vi "Example_Demo.vi"() -> ()   [LabVIEW 2017, in "maxonEPOS.lvlib"]
doc: "Example how to work with some maxon EPOS VIs. Before starts this example the device must be tuned and the parameter settings must be correct.\nThe example shows:\n - how to initialise and close an interface (with a dialog)\n - dialog shows configured parameters and data\n - enable/disable a device\n - start/stop a relative movement\n - profile and node settings\n - use of the data recorder\n - update of actual values\n\nThe example must be terminated with the button \"Exit\"!"
uses:
  maxonEPOS.lvlib
panel:
  in  "data recorder":T1={"samplingPeriod"=12, "nbOfPrecedingSamples"=0}
  out "Position Graph":i32[](graph)=[374267, 374268, 374268, 374269, 374271, 374273, 374275, 374279, 374282, 374287, 374291, 374296, 374301, 374306, 374311, 374317, 374322, 374327, 374333, 374340, 374347, 374354, 374362, 374371, 374380, 374390, 374399, 374408, 374417, 374428, 374438, 374450, 374461, 374471, 374482, 374492, 374504, 374517, 374531, 374545, 374560, 374574, 374589, 374604, 374620, 374635, 374649, 374665, 374682, 374699, 374716, 374732, 374751, 374769, 374787, 374806, 374825, 374843, 374860, 374874, 374886, 374898, 374910, 374922, 374934, 374946, 374958, 374969, 374982, 374996, 375011, 375023, 375035, 375046, 375056, 375066, 375076, 375085, 375093, 375102, 375110, 375119, 375128, 375137, 375146, 375154, 375162, 375169, 375175, 375181, 375187, 375191, 375197, 375201, 375206, 375211, 375215, 375219, 375224, 375227, 375231, 375233, 375236, 375237, 375239, 375240, 375240, 375241, 375241, 375241, 375241, 375241, 375241, 375242, 375243, 375244, 375245, 375247, 375248, 375250, 375251, 375252, 375253, 375254, 375255, 375256, 375256, 375257, 375257, 375257, 375257, 375258, 375258, 375259, 375259, 375260, 375261, 375261, 375262, 375262, 375263, 375263, 375263, 375263, 375264, 375264, 375264, 375265, 375265, 375265, 375266, 375266, 375266, 375266, 375266, 375267, 375267, 375267, 375267, 375267, 375267, 375267, 375267, 375267, 375268, 375268, 375268, 375268, 375268, 375268, 375268, 375268, 375268, 375268, 375268, 375268, 375268, 375268, 375268, 375268, 375268, 375268, 375268, 375268, 375268, 375268, 375268, 375268, 375268, 375268, 375268, 375268, 375268, 375268, 375268, 375268, 375268, 375268, 375268, 375268, 375268, 375268, 375268, 375268, 375268, 375268, 375268, 375268, 375268, 375268, 375268, 375268, 375268, 375268, 375268, 375268, 375268, 375268, 375268, 375268, 375268, 375268, 375268, 375268, 375268, 375268, 375268, 375268, 375268, 375268, 375268, 375268, 375268, 375268, 375268, 375268, 375268, 375268, 375268, 375268, 375268, 375268, 375268, 375268, 375268, 375268, 375268, 375268, 375268, 375268, 375268, 375268, 375268, 375268, 375268, 375268]
  in  "flags":cluster{"Absolute":i32, "Immediately":i32}={"Absolute"=0, "Immediately"=1} {"Immediately" items=["false", "true"]; "Absolute" items=["false", "true"]}
  out "axis data ex":T2
  out "enabled":bool=TRUE
  in  "Exit":bool
  in  "relative position":i32=1000
  in  "position profile":T3={"profileVelocity"=1000, "profileAcceleration"=10000, "profileDeceleration"=10000}
  in  "nodeId":u16=1
  in  "ShowParameters":bool
  in  "DeviceSettings":bool
  in  "MoveToPosition":bool
  in  "Halt":bool
  in  "Enable / Disable":bool
  in  "Axis":cluster{"keyHandle":u32, "nodeId":u16}
  # "EPOS2/4 Positioning Demo"
  # "Position Profile"
  # "Actual Values"
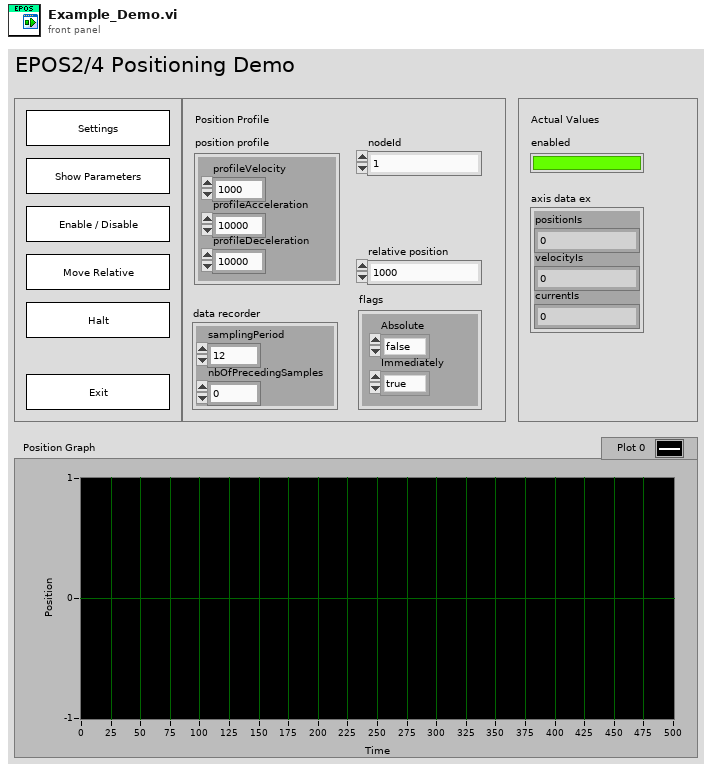
[diagram p1: front panel]
types:
  T1 = cluster{"samplingPeriod":u16, "nbOfPrecedingSamples":u16}
  T2 = cluster{"positionIs":i32, "velocityIs":i32, "currentIs":i32}
  T3 = cluster{"profileVelocity":u32, "profileAcceleration":u32, "profileDeceleration":u32}
  T4 = cluster{"Enum":enum16{"Device Settings", "Halt", "Move Position", "ShowParameters", "Enable-Disable", "Exit", "Update"}, bool}
  T5 = cluster{"recorded object 1":cluster{"objectIndex":u16, "objectSubIndex":u8, "objectSize":u8}, "recorded object 2":cluster{"objectIndex":u16, "objectSubIndex":u8, "objectSize":u8}, "recorded object 3":cluster{"objectIndex":u16, "objectSubIndex":u8, "objectSize":u8}, "recorded object 4":cluster{"objectIndex":u16, "objectSubIndex":u8, "objectSize":u8}}
  T6 = enum16{"Disabled", "Enabled", "Quickstop", "Fault"}
  T7 = enum16{"Device Settings", "Halt", "Move Position", "ShowParameters", "Enable-Disable", "Exit", "Update"}
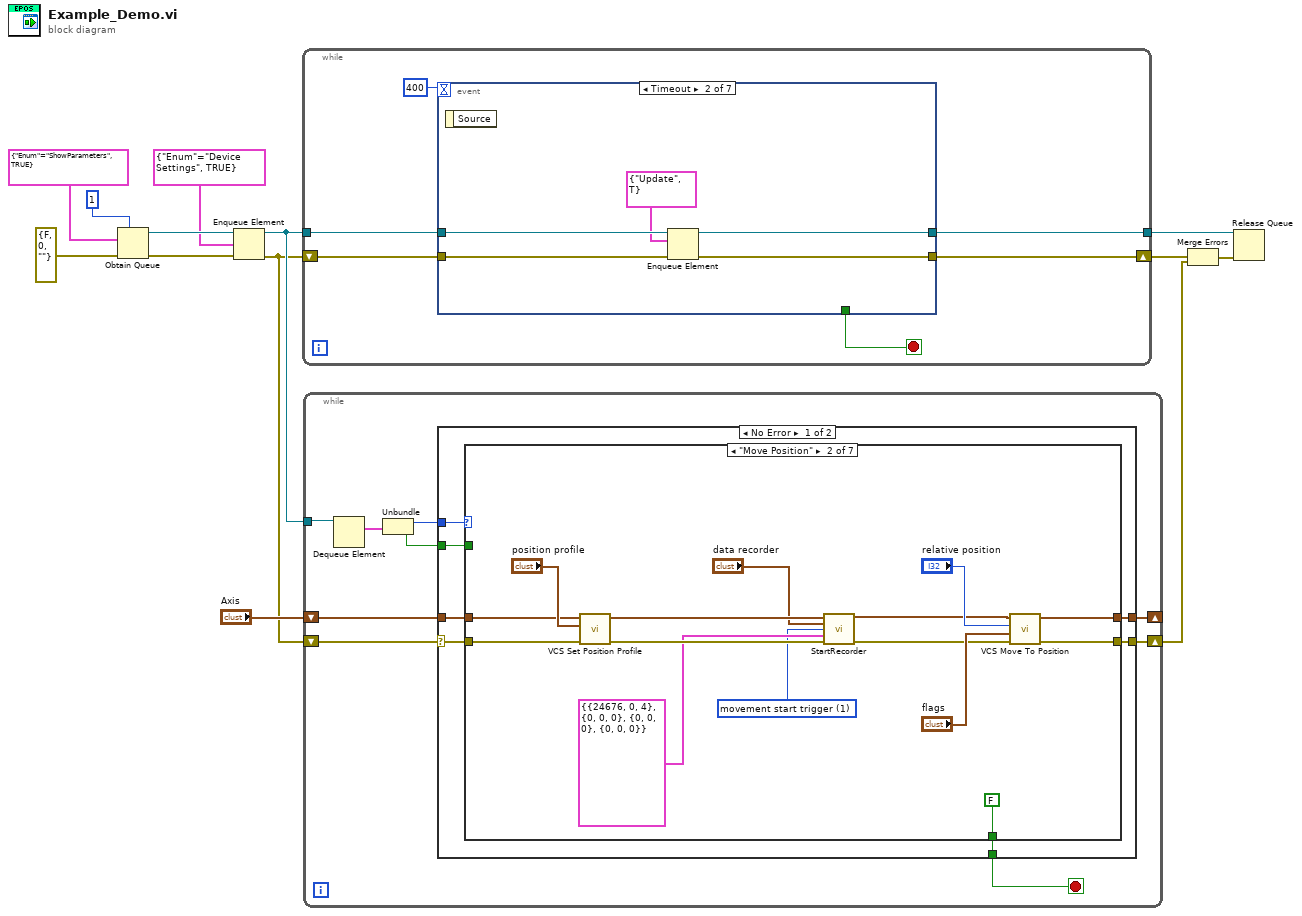
[diagram p0: block diagram]
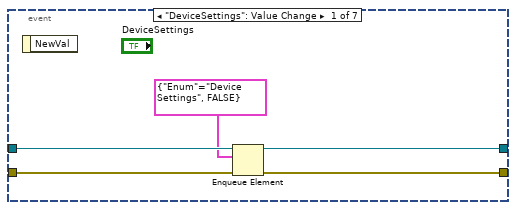
[diagram p2: hidden frame]
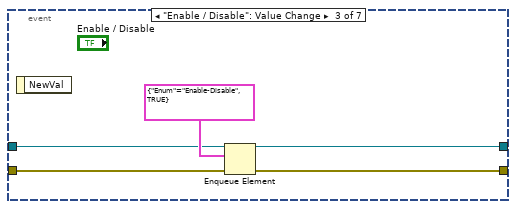
[diagram p3: hidden frame]
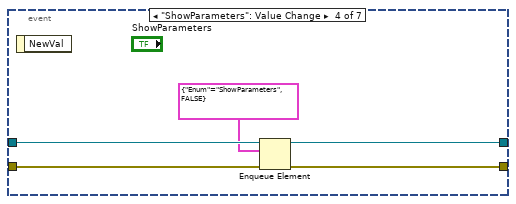
[diagram p4: hidden frame]
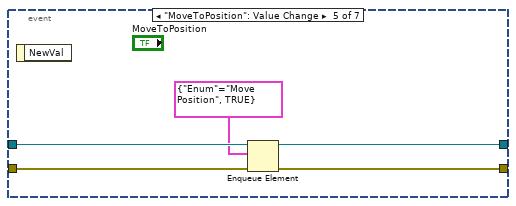
[diagram p5: hidden frame]
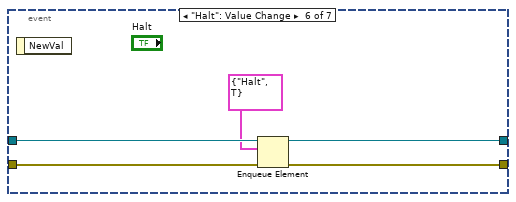
[diagram p6: hidden frame]
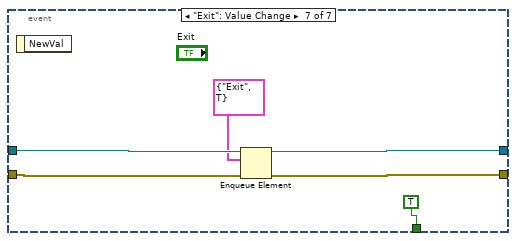
[diagram p7: hidden frame]
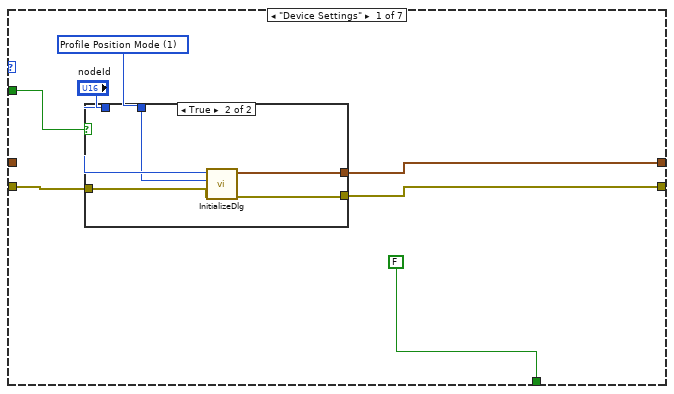
[diagram p8: hidden frame]
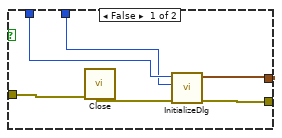
[diagram p9: hidden frame]
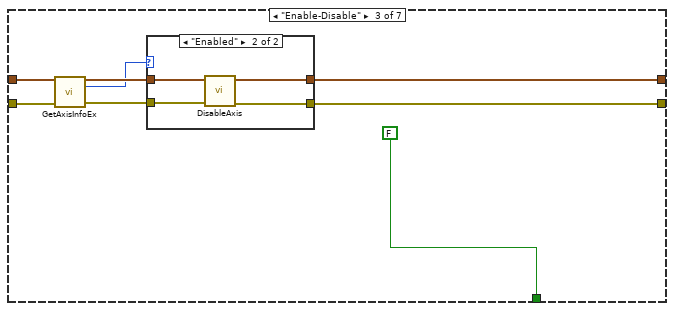
[diagram p10: hidden frame]
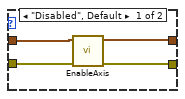
[diagram p11: hidden frame]
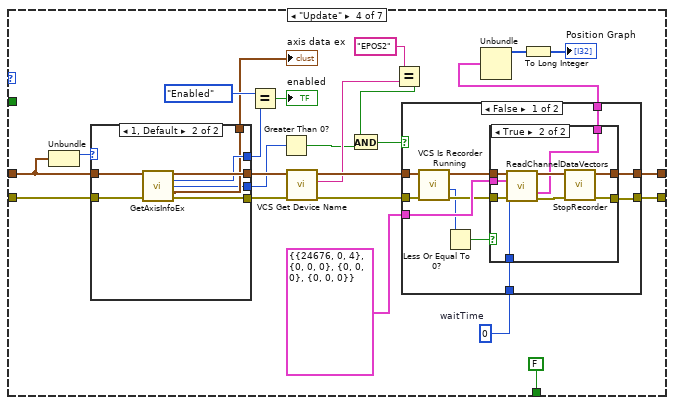
[diagram p12: hidden frame]
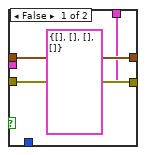
[diagram p13: hidden frame]
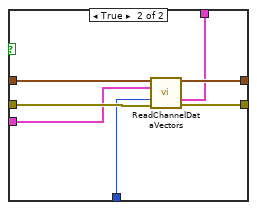
[diagram p14: hidden frame]
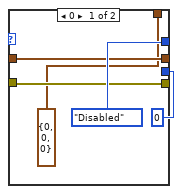
[diagram p15: hidden frame]
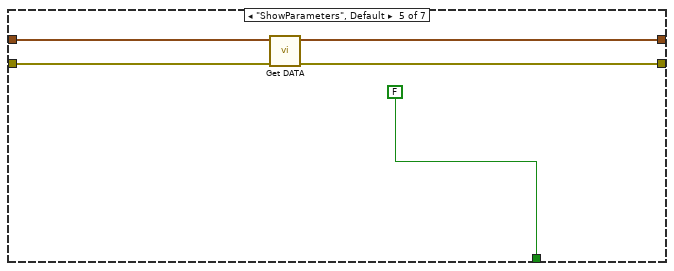
[diagram p16: hidden frame]
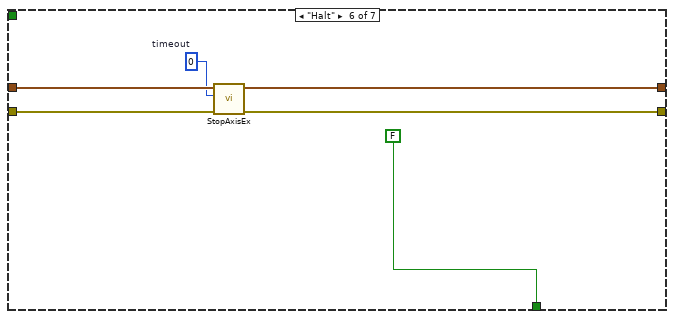
[diagram p17: hidden frame]
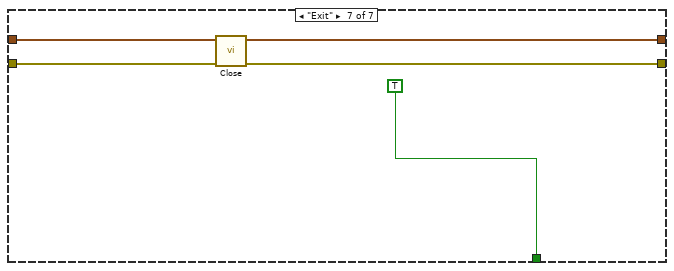
[diagram p18: hidden frame]
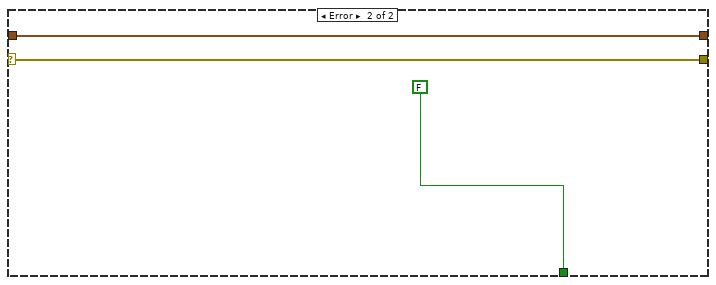
[diagram p19: hidden frame]
diagram:
  n1 = Obtain Queue(max queue size (-1, unlimited)=1 ("Maximale Queue-Größe (-1, unbegrenzt)"), element data type=T4 {"Enum"=enum."ShowParameters", TRUE}, error in (no error)=errorcluster {"status"=FALSE, "code"=0, "source"=""}) -> (queue out=w13:refnum<queue>, error out=w12:errorcluster)  [unwired: 2 in, 1 out]
  n2 = Enqueue Element(queue=w13, element=T4 {"Enum"=enum."Device Settings", TRUE}, error in (no error)=w12) -> (queue out=w6:refnum<queue>, error out=w5:errorcluster)  [unwired: 1 in, 1 out]
  n3 = while {
    tunnel: w6 -> [w19]
    tunnel: [w15] -> w9
    shift-right: [w14] -> w4
    shift-left: w5 -> [w18]
    stop <- w17 stop-if-true
    n4 = event shown="[1] Timeout" {
      selector: _ -> [_ _ _ _ _ _ _]
      dyn-events: _ -> [_ _ _ _ _ _ _]
      timeout: 400 -> [_ _ _ _ _ _ _]
      tunnel: w19 -> [w24 w26 w30 w39 w44 w49 w54]
      tunnel: w18 -> [w23 w29 w34 w38 w43 w48 w53]
      tunnel: [w22 w28 w33 w37 w42 w46 w52] -> w14
      tunnel: [_ _ _ _ _ _ TRUE] -> w17
      tunnel: [w21 w27 w32 w36 w40 w47 w51] -> w15
      event "DeviceSettings": Value Change {
        n5 = event-data() -> ()  [unwired: 1 in, 1 out]
        n6 = Enqueue Element(queue=w24, element=T4 {"Enum"=enum."Device Settings", FALSE}, error in (no error)=w23) -> (queue out=w21:refnum<queue>, error out=w22:errorcluster)  [unwired: 1 in, 1 out]
      }
      event Timeout {
        n7 = event-data() -> ()  [unwired: 1 in, 1 out]
        n8 = Enqueue Element(queue=w26, element=T4 {"Enum"=enum."Update", TRUE}, error in (no error)=w29) -> (queue out=w27:refnum<queue>, error out=w28:errorcluster)  [unwired: 1 in, 1 out]
      }
      event "Enable / Disable": Value Change {
        n9 = event-data() -> ()  [unwired: 1 in, 1 out]
        n10 = Enqueue Element(queue=w30, element=T4 {"Enum"=enum."Enable-Disable", TRUE}, error in (no error)=w34) -> (queue out=w32:refnum<queue>, error out=w33:errorcluster)  [unwired: 1 in, 1 out]
      }
      event "ShowParameters": Value Change {
        n11 = event-data() -> ()  [unwired: 1 in, 1 out]
        n12 = Enqueue Element(queue=w39, element=T4 {"Enum"=enum."ShowParameters", FALSE}, error in (no error)=w38) -> (queue out=w36:refnum<queue>, error out=w37:errorcluster)  [unwired: 1 in, 1 out]
      }
      event "MoveToPosition": Value Change {
        n13 = event-data() -> ()  [unwired: 1 in, 1 out]
        n14 = Enqueue Element(queue=w44, element=T4 {"Enum"=enum."Move Position", TRUE}, error in (no error)=w43) -> (queue out=w40:refnum<queue>, error out=w42:errorcluster)  [unwired: 1 in, 1 out]
      }
      event "Halt": Value Change {
        n15 = event-data() -> ()  [unwired: 1 in, 1 out]
        n16 = Enqueue Element(queue=w49, element=T4 {"Enum"=enum."Halt", TRUE}, error in (no error)=w48) -> (queue out=w47:refnum<queue>, error out=w46:errorcluster)  [unwired: 1 in, 1 out]
      }
      event "Exit": Value Change {
        n17 = event-data() -> ()  [unwired: 1 in, 1 out]
        n18 = Enqueue Element(queue=w54, element=T4 {"Enum"=enum."Exit", TRUE}, error in (no error)=w53) -> (queue out=w51:refnum<queue>, error out=w52:errorcluster)  [unwired: 1 in, 1 out]
      }
    }
  }
  n19 = while {
    shift-right: [w63] -> _
    shift-left: "Axis" -> [w59]
    shift-right: [w64] -> w2
    shift-left: w5 -> [w58]
    tunnel: w6 -> [w62]
    stop <- w57 stop-if-true
    n20 = Dequeue Element(queue=w62) -> (element=w56:T4)  [unwired: 2 in, 3 out]
    n21 = Unbundle(w56) -> ("Enum"=w61:T7, w60:bool)
    n22 = case shown="No Error" w58 {
      selector: w58 -> [w66 w204]
      tunnel: [w71 w204] -> w64
      tunnel: [w70 w203] -> w63
      tunnel: w61 -> [w65 _]
      tunnel: w60 -> [w69 _]
      tunnel: [w68 FALSE] -> w57
      tunnel: w59 -> [w67 w203]
      frame No Error {
        n23 = case shown="\"Move Position\"" w65 {
          tunnel: [w77 w99 w106 w136 w189 w194 w202] -> w71
          tunnel: [w78 w100 w105 w137 w188 w195 w199] -> w70
          tunnel: w69 -> [w72 _ _ _ _ _ _]
          tunnel: [FALSE FALSE FALSE FALSE FALSE FALSE TRUE] -> w68
          tunnel: w66 -> [w73 w90 w108 w141 w190 w196 w200]
          tunnel: w67 -> [_ w91 w109 w142 w191 w197 w199]
          frame "Device Settings" {
            w75 = i8 1 items=["Profile Position Mode"=1, "Profile Velocity Mode"=3, "Homing Mode"=6, "Interpolated Position Mode"=7, "Position Mode"=-1, "Velocity Mode"=-2, "Current Mode"=-3, "Master Encoder Mode"=-5, "Step Direction Mode"=-6] ("modes of operations")
            n24 = case shown="True" w72 {
              tunnel: [w82 w89] -> w78
              tunnel: [w83 w88] -> w77
              tunnel: "nodeId" -> [w81 w87]
              tunnel: w75 -> [w80 w86]
              tunnel: w73 -> [w79 w85]
              frame False {
                n25 = call "Close.vi"("error in (no error)"=w79) -> ("error out"=w84:errorcluster)  [unwired: 10 in]
                n26 = call "InitializeDlg.vi"("error in (no error)"=w84, "modes of operations"=w80, "nodeId"=w81) -> ("error out"=w83:errorcluster, "axis out"=w82:cluster{"keyHandle":u32, "nodeId":u16})  [unwired: 7 in]
              }
              frame True {
                n27 = call "InitializeDlg.vi"("error in (no error)"=w85, "modes of operations"=w86, "nodeId"=w87) -> ("error out"=w88:errorcluster, "axis out"=w89:cluster{"keyHandle":u32, "nodeId":u16})  [unwired: 7 in]
              }
            }
          }
          frame "Move Position" {
            w94 = u8 1 items=["movement start trigger"=1, "error trigger"=2, "digital input trigger"=4, "movement end trigger"=8] ("trigger type")
            n28 = call "VCS Set Position Profile.vi"("error in (no error)"=w90, "position profile"="position profile", "axis in"=w91) -> ("error out"=w96:errorcluster, "axis out"=w93:cluster{"keyHandle":u32, "nodeId":u16})  [unwired: 7 in]
            n29 = call "StartRecorder.vi"("axis in"=w93, "parameter"="data recorder", "trigger type"=w94, "recorded objects"=T5 {"recorded object 1"={"objectIndex"=24676, "objectSubIndex"=0, "objectSize"=4}, "recorded object 2"={"objectIndex"=0, "objectSubIndex"=0, "objectSize"=0}, "recorded object 3"={"objectIndex"=0, "objectSubIndex"=0, "objectSize"=0}, "recorded object 4"={"objectIndex"=0, "objectSubIndex"=0, "objectSize"=0}}, "error in (no error)"=w96) -> ("axis out"=w98:cluster{"keyHandle":u32, "nodeId":u16}, "error out"=w97:errorcluster)  [unwired: 9 in]
            n30 = call "VCS Move To Position.vi"("error in (no error)"=w97, "flags"="flags", "targetPosition"="relative position", "axis in"=w98) -> ("error out"=w99:errorcluster, "axis out"=w100:cluster{"keyHandle":u32, "nodeId":u16})  [unwired: 6 in]
          }
          frame "Enable-Disable" {
            n31 = call "GetAxisInfoEx.vi"("axis in"=w109, "error in (no error)"=w108) -> ("axis out"=w110:cluster{"keyHandle":u32, "nodeId":u16}, "axis state"=w107:T6, "error out"=w111:errorcluster)  [unwired: 9 in, 2 out]
            n32 = case shown="\"Enabled\"" w107 {
              tunnel: w111 -> [w115 w120]
              tunnel: w110 -> [w116 w118]
              tunnel: [w113 w119] -> w106
              tunnel: [w114 w117] -> w105
              frame "Disabled", Default {
                n33 = call "EnableAxis.vi"("error in (no error)"=w115, "axis in"=w116) -> ("error out"=w113:errorcluster, "axis out"=w114:cluster{"keyHandle":u32, "nodeId":u16})  [unwired: 4 in]
              }
              frame "Enabled" {
                n34 = call "DisableAxis.vi"("error in (no error)"=w120, "axis in"=w118) -> ("error out"=w119:errorcluster, "axis out"=w117:cluster{"keyHandle":u32, "nodeId":u16})  [unwired: 4 in]
              }
            }
          }
          frame "Update" {
            w121 = u32 0  # waitTime
            n35 = Unbundle(w142) -> ("keyHandle"=w143:u32)  [unwired: 1 out]
            n36 = case shown="1, Default" w143 {
              tunnel: [w179 w186] -> w131
              tunnel: [w178 w187] -> w134
              tunnel: [T6."Disabled" ("axis state") w185] -> w145
              tunnel: w142 -> [w179 w184]
              tunnel: w141 -> [w178 w183]
              tunnel: [T2 {"positionIs"=0, "velocityIs"=0, "currentIs"=0} ("axis data") w182] -> w139
              tunnel: [0 ("targetReached") w181] -> w128
              frame 0 {
              }
              frame 1, Default {
                n37 = call "GetAxisInfoEx.vi"("axis in"=w184, "error in (no error)"=w183) -> ("axis out"=w186:cluster{"keyHandle":u32, "nodeId":u16}, "axis state"=w185:T6, "targetReached"=w181:i32, "axis data ex"=w182:T2, "error out"=w187:errorcluster)  [unwired: 9 in]
              }
            }
            "axis data ex" <- w139
            n38 = Equal?(x=T6."Enabled" ("axis state"), y=w145) -> (x = y?=→"enabled":bool)
            n39 = Greater Than 0?(x=w128) -> (x > 0?=w127:bool)
            n40 = call "VCS Get Device Name.vi"("error in (no error)"=w134, "axis in"=w131) -> ("error out"=w133:errorcluster, "deviceName"=w129:string, "axis out"=w132:cluster{"keyHandle":u32, "nodeId":u16})  [unwired: 7 in]
            n41 = Equal?(x="EPOS2", y=w129) -> (x = y?=w126:bool)
            n42 = And(x=w126, y=w127) -> (x .and. y?=w125:bool)
            n43 = case shown="False" w125 {
              tunnel: w132 -> [w150 w175]
              tunnel: w133 -> [w153 w174]
              tunnel: [w155 w173] -> w137
              tunnel: [w156 w172] -> w136
              tunnel: T5 {"recorded object 1"={"objectIndex"=24676, "objectSubIndex"=0, "objectSize"=4}, "recorded object 2"={"objectIndex"=0, "objectSubIndex"=0, "objectSize"=0}, "recorded object 3"={"objectIndex"=0, "objectSubIndex"=0, "objectSize"=0}, "recorded object 4"={"objectIndex"=0, "objectSubIndex"=0, "objectSize"=0}} ("recorded objects") -> [w154 w171]
              tunnel: [w146 w170] -> w122
              tunnel: w121 -> [w147 w169]
              frame False {
                n44 = call "VCS Is Recorder Running.vi"("error in (no error)"=w153, "axis in"=w150) -> ("error out"=w152:errorcluster, "isRunning"=w149:i32, "axis out"=w151:cluster{"keyHandle":u32, "nodeId":u16})  [unwired: 7 in]
                n45 = Less Or Equal To 0?(x=w149) -> (x <= 0?=w148:bool)
                n46 = case shown="True" w148 {
                  tunnel: [w159 w162] -> w156
                  tunnel: [w158 w161] -> w155
                  tunnel: w154 -> [_ w168]
                  tunnel: w152 -> [w159 w167]
                  tunnel: w151 -> [w158 w166]
                  tunnel: w147 -> [_ w165]
                  tunnel: [cluster{u32[], u32[], u32[], u32[]} {[], [], [], []} ("U32 data vectors") w160] -> w146
                  frame False {
                  }
                  frame True {
                    n47 = call "ReadChannelDataVectors.vi"("axis in"=w166, "recorded objects"=w168, "waitBeforeRead"=w165, "error in (no error)"=w167) -> ("axis out"=w164:cluster{"keyHandle":u32, "nodeId":u16}, "U32 data vectors"=w160:cluster{u32[], u32[], u32[], u32[]}, "error out"=w163:errorcluster)  [unwired: 7 in, 2 out]
                    n48 = call "StopRecorder.vi"("error in (no error)"=w163, "axis in"=w164) -> ("error out"=w162:errorcluster, "axis out"=w161:cluster{"keyHandle":u32, "nodeId":u16})  [unwired: 4 in]
                  }
                }
              }
              frame True {
                n49 = call "ReadChannelDataVectors.vi"("axis in"=w175, "recorded objects"=w171, "waitBeforeRead"=w169, "error in (no error)"=w174) -> ("axis out"=w173:cluster{"keyHandle":u32, "nodeId":u16}, "U32 data vectors"=w170:cluster{u32[], u32[], u32[], u32[]}, "error out"=w172:errorcluster)  [unwired: 7 in, 2 out]
              }
            }
            n50 = Unbundle(w122) -> (w123:u32[])  [unwired: 3 out]
            n51 = To Long Integer(number=w123) -> (32bit integer=→"Position Graph":i32[])
          }
          frame "ShowParameters", Default {
            n52 = call "Get DATA.vi"("error in"=w190, "axis in"=w191) -> ("error out"=w189:errorcluster, "axis out"=w188:cluster{"keyHandle":u32, "nodeId":u16})  [unwired: 8 in]
          }
          frame "Halt" {
            w193 = u32 0  # timeout
            n53 = call "StopAxisEx.vi"("error in (no error)"=w196, "timeout"=w193, "axis in"=w197) -> ("error out"=w194:errorcluster, "axis out"=w195:cluster{"keyHandle":u32, "nodeId":u16})  [unwired: 3 in]
          }
          frame "Exit" {
            n54 = call "Close.vi"("error in (no error)"=w200) -> ("error out"=w202:errorcluster)  [unwired: 10 in]
          }
        }
      }
      frame Error {
      }
    }
  }
  n55 = Merge Errors(w4, w2) -> (w3:errorcluster)
  n56 = Release Queue(queue=w9, error in (no error)=w3) -> ()  [unwired: 1 in, 3 out]
